vi "vision_webcam_V2_external_no_queue.vi"(11 "dup Message Queue 2":refnum<queue>) -> ()   [LabVIEW 2017]
uses:
  UI Error Handlers/support/Message Queue/Message Cluster.ctl
  <vilib>/userdefined/High Color/IMAQdx.ctl
  <vilib>/vision/Avi.llb/IMAQ AVI2 Refnum.ctl
  Globals/Global - Configuration Options.vi
  Globals/Global - All RT Loop Stop.vi
  <vilib>/vision/driver/NI_Vision_Acquisition_Software.lvlib
  UI Error Handlers/support/Message Queue/Message Queue.lvlib
panel:
  out "Webcam":T1(plugin-control)
  out "concatenated string 4":string
  out "x-y":u32
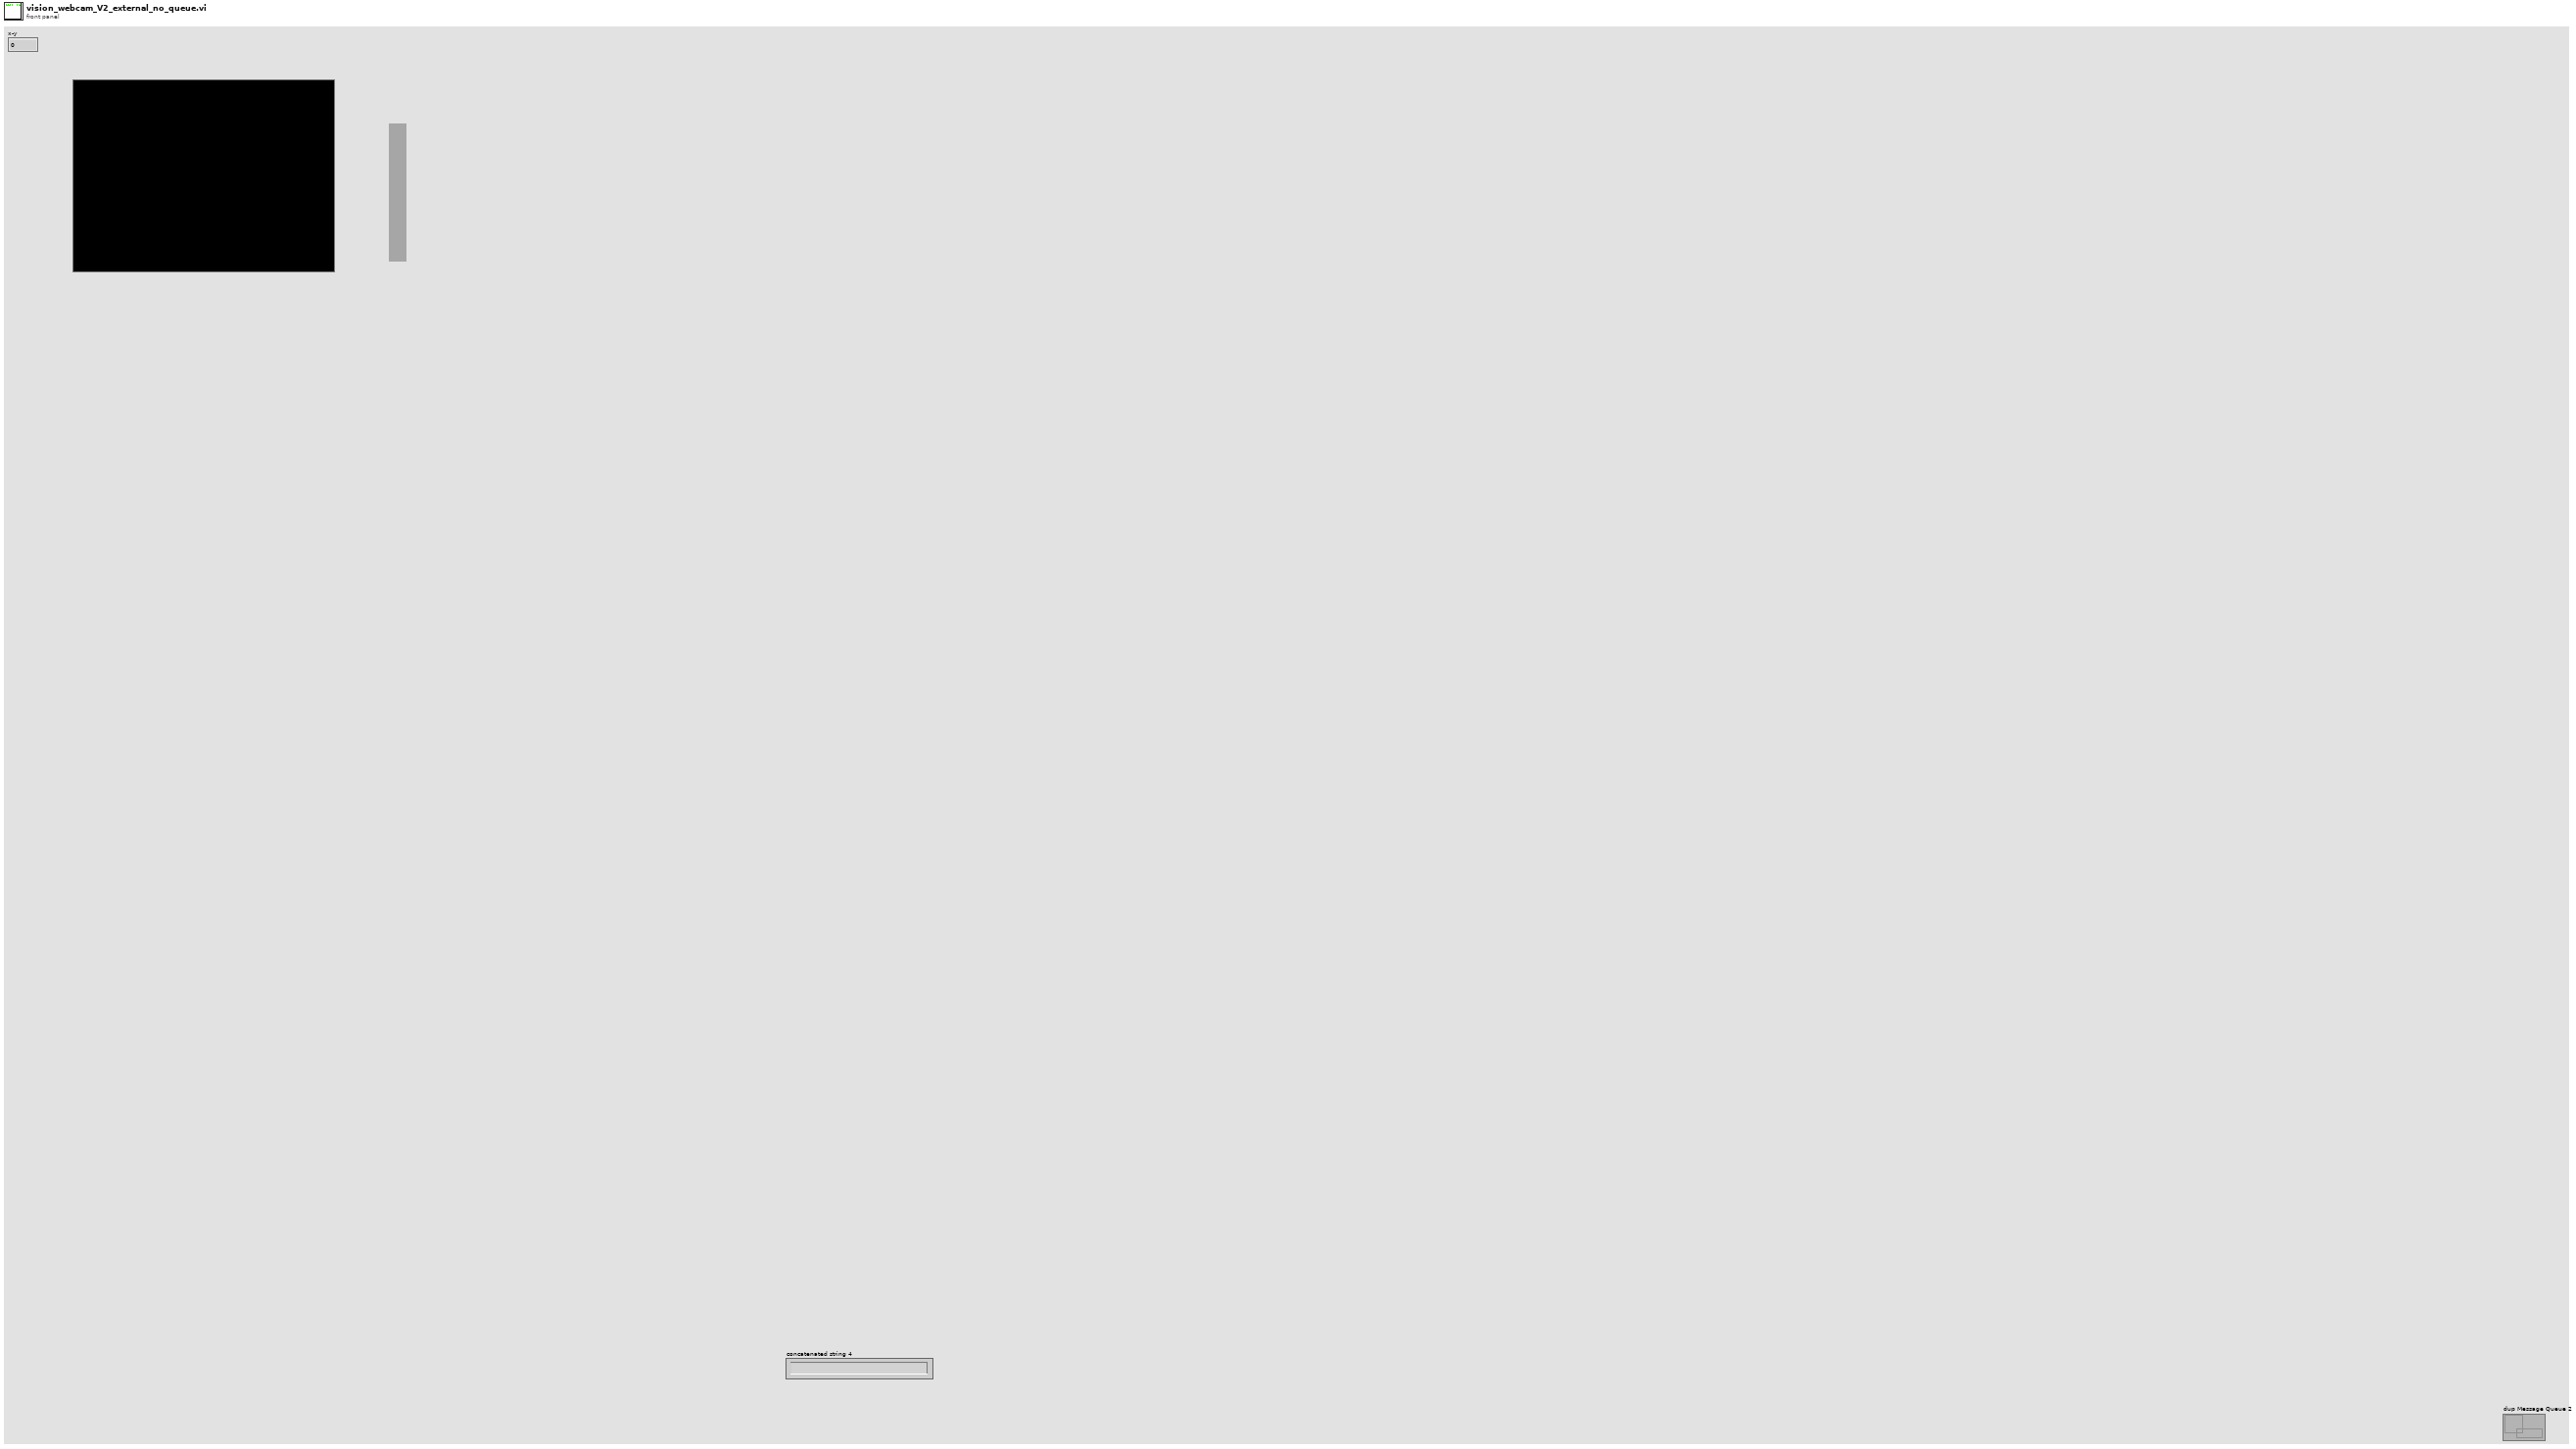
[diagram p1: front panel]
types:
  T1 = typedef "IMAQ Image.ctl" = refnum<image>
  T2 = typedef "IMAQ AVI2 Refnum.ctl" = refnum<k20>
  T3 = typedef "IMAQdx.ctl" = refnum<k21>
  T4 = typedef "Image Type" = u32
  T5 = cluster{"Tool data":cluster{"Number of teeth":sgl}, "Cutting data":cluster{"rpm":sgl}, "Limits":cluster{"Magnitude threshold":sgl, "Tolerance":sgl}, "G1 status":cluster{"G1 trigger":bool}}
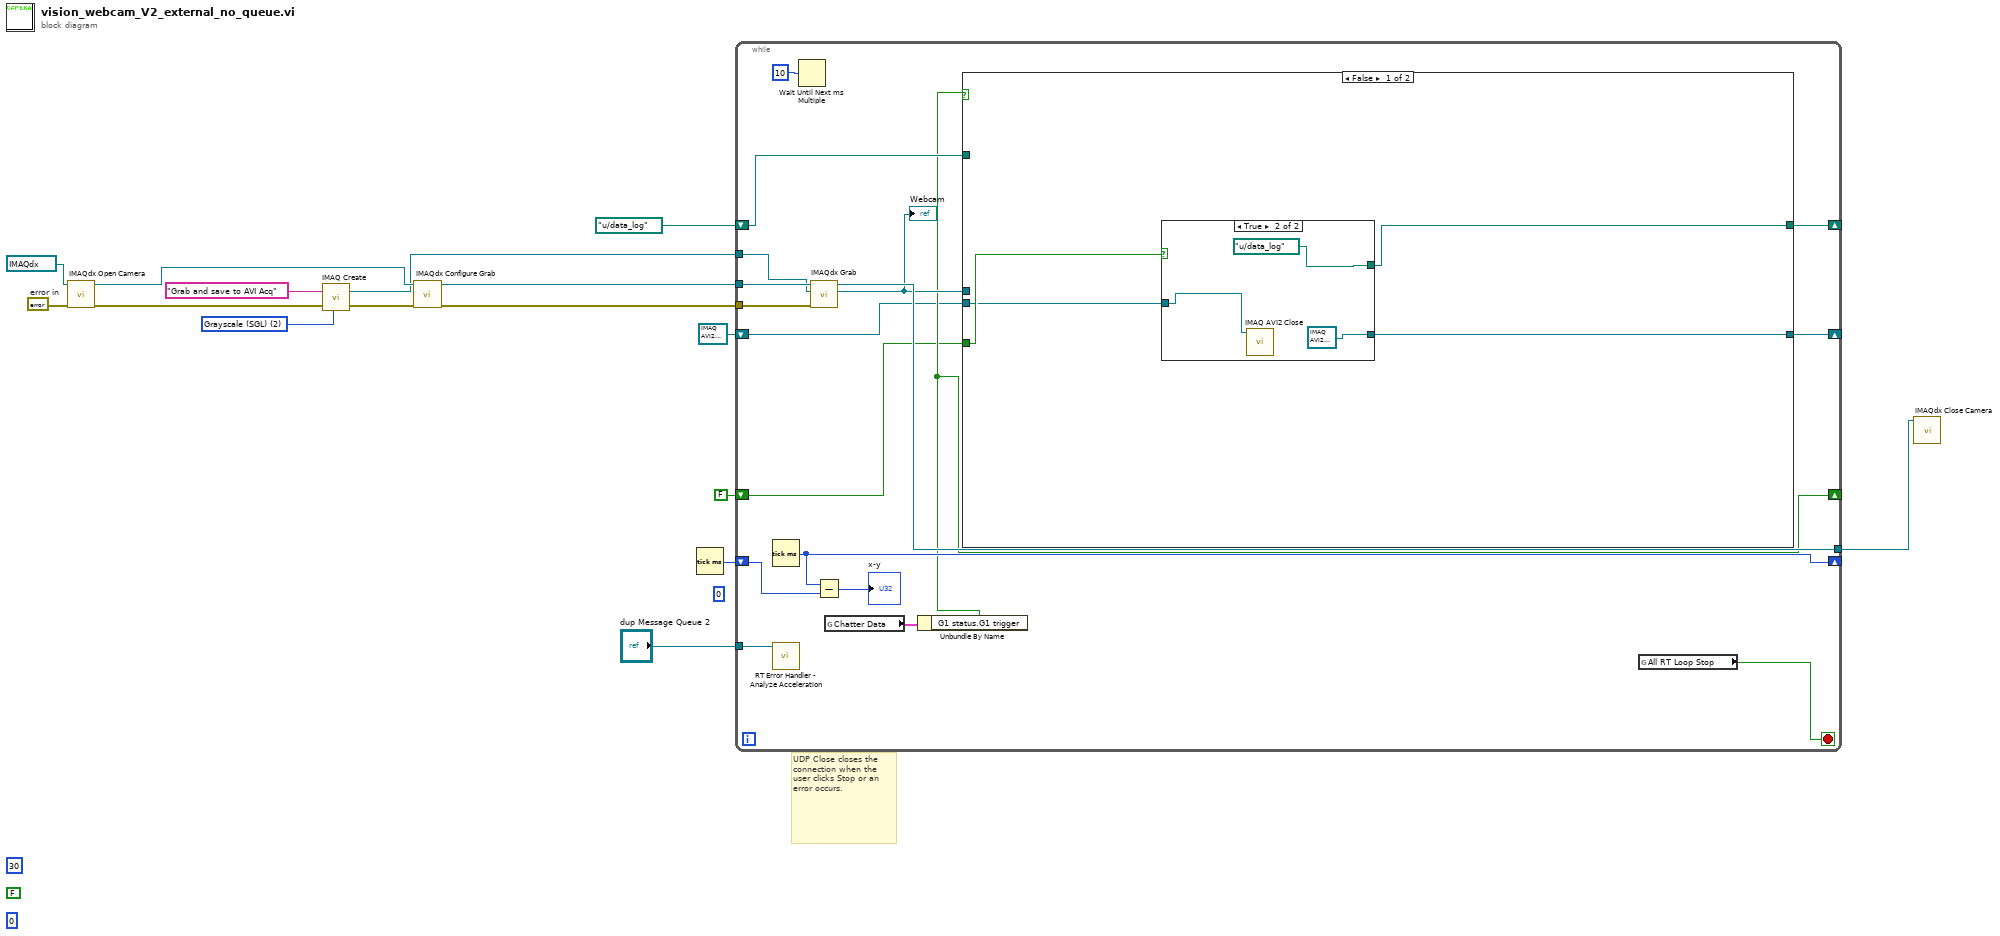
[diagram p0: block diagram]
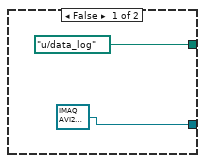
[diagram p2: hidden frame]
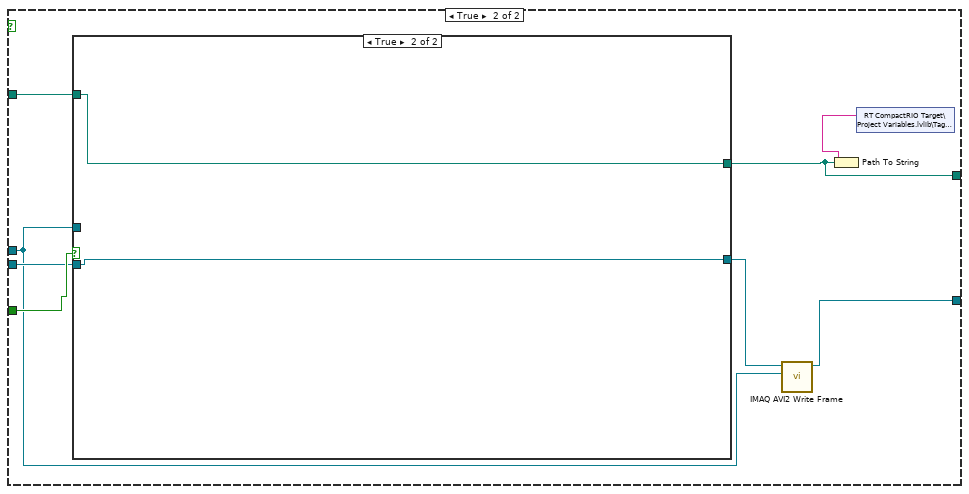
[diagram p3: hidden frame]
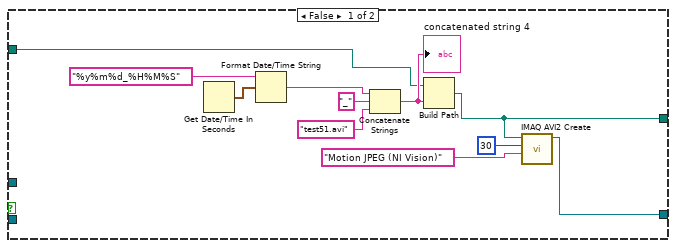
[diagram p4: hidden frame]
diagram:
  (unwired) 0
  w11 = T4 2 items=["Grayscale (U8)", "Grayscale (I16)", "Grayscale (SGL)", "Complex (CSG)", "RGB (U32)", "HSL (U32)", "RGB (U64)", "Grayscale (U16)"] ("Image Type")
  (unwired) u32 30 ("Frames Per Second")
  w12 = errorcluster {"status"=FALSE, "code"=0, "source"=""}  # error in
  (unwired) i16 0 ("A(I16) 11")
  (unwired) FALSE
  # "UDP Close closes the connection when the user clicks Stop or an error occurs."
  n1 = call <vilib>:"IMAQdx Open Camera.vi"("error in"=w12, "Session In"=T3 "cam1") -> ("error out"=w10:errorcluster, "Session Out"=w14:T3)  [unwired: 8 in]
  n2 = call "IMAQ Create"("Image Name"="Grab and save to AVI Acq", "Image Type"=w11, "error in (no error)"=w10) -> ("New Image"=w7:T1, "error out"=w6:errorcluster)  [unwired: 2 in]
  n3 = call <vilib>:"IMAQdx Configure Grab.vi"("error in"=w6, "Session In"=w14) -> ("error out"=w5:errorcluster, "Session Out"=w8:T3)  [unwired: 8 in]
  n4 = Tick Count (ms)() -> (millisecond timer value=w15:u32)
  n5 = while {
    tunnel: "dup Message Queue 2" -> [w34]
    shift-right: [w30] -> _
    shift-left: w15 -> [w31]
    tunnel: w8 -> [w29]
    tunnel: w7 -> [w28]
    tunnel: w5 -> [w27]
    tunnel: [w26] -> w1
    shift-right: [w21] -> _
    shift-left: path "u:/data_log" ("AVI Path") -> [w22]
    shift-right: [w20] -> _
    shift-left: FALSE ("G1 trigger") -> [w19]
    shift-right: [w17] -> _
    shift-left: T2 refnum ("AVI Refnum") -> [w18]
    stop <- w24 stop-if-true
    n6 = Tick Count (ms)() -> (millisecond timer value=w30:u32)
    n7 = call "RT Error Handler - Analyze Acceleration.vi"("Message Queue"=w34) -> ()  [unwired: 10 in, 1 out]
    n8 = Wait Until Next ms Multiple(millisecond multiple=u32 10) -> ()  [unwired: 1 out]
    n9 = call <vilib>:"IMAQdx Grab.vi"("error in"=w27, "Image In"=w28, "Session In"=w29) -> ("Image Out"=w23:T1, "Session Out"=w26:T3)  [unwired: 5 in, 2 out]
    "Webcam" <- w23
    n10 = Subtract(x=w30, y=w31) -> (x-y=→"x-y":u32)
    n11 = global read "Global - Configuration Options.vi" "Chatter Data"() -> (w33:T5)
    n12 = Unbundle By Name(w33) -> ("G1 status.G1 trigger"=w20:bool)
    n13 = case shown="False" w20 {
      tunnel: w23 -> [_ w45]
      tunnel: w22 -> [_ w50]
      tunnel: [w38 w49] -> w21
      tunnel: w19 -> [w37 w48]
      tunnel: w18 -> [w36 w47]
      tunnel: [w35 w44] -> w17
      frame False {
        n14 = case shown="True" w37 {
          tunnel: [path "u:/data_log" ("AVI Path") path "u:/data_log" ("AVI Path")] -> w38
          tunnel: w36 -> [_ w41]
          tunnel: [T2 refnum ("AVI Refnum") T2 refnum ("AVI Refnum")] -> w35
          frame False {
          }
          frame True {
            n15 = call "IMAQ AVI2 Close"("AVI Refnum"=w41) -> ()  [unwired: 10 in, 1 out]
          }
        }
      }
      frame True {
        n16 = case shown="True" w48 {
          tunnel: w45 -> [_ _]
          tunnel: [w54 w64] -> w49
          tunnel: w50 -> [w53 w64]
          tunnel: [w52 w63] -> w46
          tunnel: w47 -> [_ w63]
          frame False {
            n17 = Get Date/Time In Seconds() -> (seconds since 1Jan1904=w60:timestamp)
            n18 = Format Date/Time String(time format string (%c)="%y%m%d_%H%M%S", seconds (now)=w60) -> (date/time string=w61:string)  [unwired: 1 out]
            n19 = Concatenate Strings(w61, "_" ("string"), "test51.avi" ("name or relative path")) -> (w62:string)
            "concatenated string 4" <- w62
            n20 = Build Path(base path=w53, name or relative path=w62) -> (appended path=w54:path)
            n21 = call "IMAQ AVI2 Create"("Codec"="Motion JPEG (NI Vision)", "Frames Per Second"=u32 30, "AVI Path"=w54) -> ("AVI Refnum"=w52:T2)  [unwired: 7 in, 1 out]
          }
          frame True {
          }
        }
        n22 = call "IMAQ AVI2 Write Frame"("Image"=w45, "AVI Refnum"=w46) -> ("AVI Refnum (duplicate)"=w44:T2)  [unwired: 7 in, 2 out]
        n23 = Path To String(path=w49) -> (string=w51:string)
        n24 = shared-variable "RT CompactRIO Target\\Project Variables.lvlib\\Tag Video"(w51) -> ()  [unwired: 1 in, 1 out]
      }
    }
    n25 = global read "Global - All RT Loop Stop.vi" "All RT Loop Stop"() -> (w24:bool)
  }
  n26 = call <vilib>:"IMAQdx Close Camera.vi"("Session In"=w1) -> ()  [unwired: 10 in, 1 out]
